vi "subscribe command.vi"(0 "variable":string) -> (1 "IP":string, 2 "port":string, 3 "subscribe command":string)   [LabVIEW 2013]
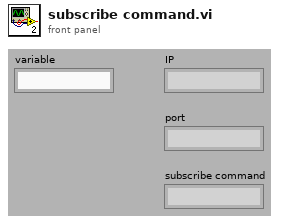
[diagram p1: front panel]
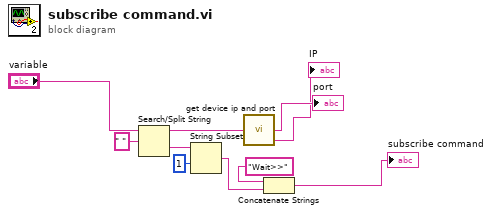
[diagram p0: block diagram]
diagram:
  n1 = Search/Split String(string="variable", search string/char (-)=" ") -> (substring before match=w5:string, match + rest of string=w2:string)  [unwired: 1 in, 1 out]
  n2 = String Subset(string=w2, offset (0)=1) -> (substring=w7:string)  [unwired: 1 in]
  n3 = call "get device ip and port.vi"("variable1"=w5) -> ("port"=→"port":string, "IP"=→"IP":string)  [unwired: 1 out]
  n4 = Concatenate Strings("Wait>>" ("search string/char (-)"), w7) -> (→"subscribe command":string)
